vi "ROI grp-Case-Sort groups table.vi"(8 "error in (no error)":errorcluster) -> (0 "error out":errorcluster)   [LabVIEW 2017]
uses:
  Globals/gl_ROI grp window globals.vi
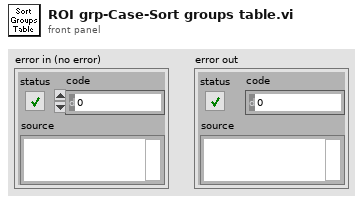
[diagram p1: front panel]
types:
  T1 = typedef "ROI grp-window ctrl refs.ctl" = cluster{"This VI":refnum<vi>, "Pane":refnum<vi>, "Table":refnum<vi>}
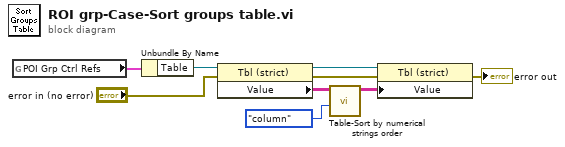
[diagram p0: block diagram]
diagram:
  n1 = global read "gl_ROI grp window globals.vi" "POI Grp Ctrl Refs"() -> (w1:T1)
  n2 = Unbundle By Name(w1) -> ("Table"=w6:refnum<vi>)
  n3 = property on="Property Node" class="Tbl (strict)"(reference=w6, error in="error in (no error)") -> (reference out=w2:refnum<vi>, error out=w9:errorcluster, "Value"=w5:string[][])
  n4 = call <userlib>:"Table-Sort by numerical strings order.vi"("Sort By in"=enum16{"row", "column"}."column", "Numerical strings table in"=w5) -> ("Sorted numerical strings table"=w4:string[][])  [unwired: 8 in, 1 out]
  n5 = property on="Property Node" class="Tbl (strict)"(reference=w2, error in=w9, "Value"=w4) -> (error out=→"error out":errorcluster)  [unwired: 1 out]
